vi "BT Rx Test Get Default Parameters.vi"(8 "error in (no error)":errorcluster, 11 "Rx Test in":refnum<class "niDTS BT Rx Test.lvclass">) -> (0 "error out":errorcluster, 2 "Parameters":T1={"Channel"=3, "Dut Tx Power"=0.0, "External Attenuation (dB)"=[0.0], "Data Rate"=enum."1", "Packet type"=enum."DH1", "Payload Data"=enum."PN9", "Carrier Mode"=enum."Burst", "Number of Packets"=1500, "Report Period (ms)"=1000.0, "BD ADDRESS"=0, "Dirty Tx"=FALSE, "Corrupt Alternate CRC"=FALSE, "Packet Header"={"LT Address"=0, "Flow"=0, "ARQN"=enum."NAK", "Sequence Bit"=0}, "Payload Header"={"LCh"=0, "HeaderFlowControlBit"=FALSE, "Length (-1 AutoSet Max)"=-1}, "Trigger"={"TriggerEdge"=enum."RISing", "TriggerSource"=enum."IMMediate", "TriggerDelay (sec)"=0.0, "TriggerTimeout (sec)"=0.0}} {"BD ADDRESS" max=16777215 format="%.0x"}, 3 "Rx Test out":refnum<class "niDTS BT Rx Test.lvclass">)   [LabVIEW 2015, in "niDTS BT.lvlib" / "niDTS BT Rx Test.lvclass"]
uses:
  niDTS BT Rx Test.lvclass
  Includes/niDTS BT Rx Test INC Parameters.ctl
  Includes/niDTS BT INC Packet Type.ctl
  Tx Test/Includes/niDTS BT Tx Test INC BD Payload Data.ctl
  Includes/niDTS BT Rx Test INC Carrier Mode.ctl
  Includes/niDTS BT Rx Test INC Packet Header.ctl
  Includes/niDTS BT Rx Test INC Payload Header.ctl
  Includes/niDTS BT DUT INC SG Trigger.ctl
  niDTS BT Rx Test.lvclass/niDTS BT Rx Test.ctl
  Includes/niDTS BT INC Standard.ctl
  niDTS BT.lvlib
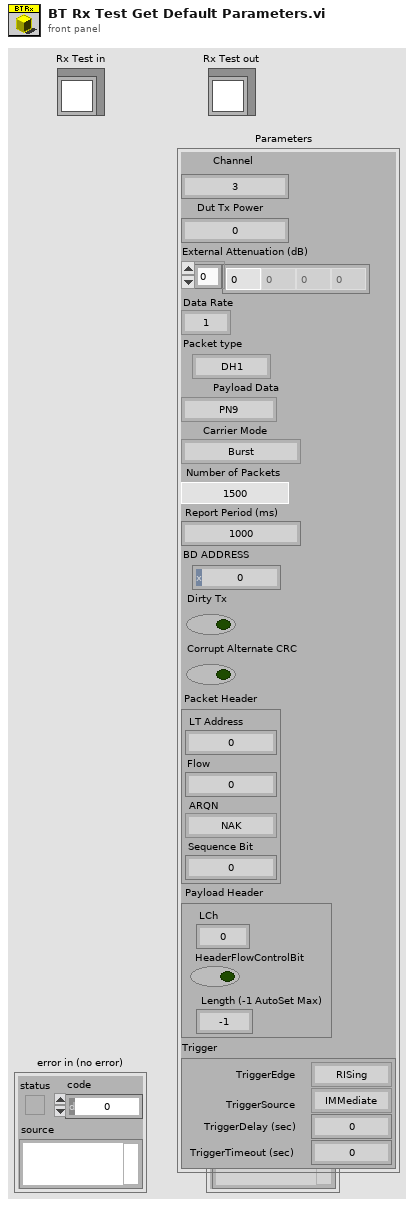
[diagram p1: front panel]
types:
  T1 = typedef "niDTS BT.lvlib/niDTS BT Rx Test INC Parameters.ctl" = cluster{"Channel":i32, "Dut Tx Power":dbl, "External Attenuation (dB)":dbl[], "Data Rate":enum16{"1", "2", "3"}, "Packet type":T2, "Payload Data":T3, "Carrier Mode":T4, "Number of Packets":i32, "Report Period (ms)":dbl, "BD ADDRESS":i64, "Dirty Tx":bool, "Corrupt Alternate CRC":bool, "Packet Header":T5, "Payload Header":T6, "Trigger":T7}
  T2 = typedef "niDTS BT.lvlib/niDTS BT INC Packet Type.ctl" = enum16{"NULL", "POLL", "FHS", "DM1", "DH1", "HV1", "HV2", "HV3", "EV3", "DV", "AUX1", "DM3", "DH3", "EV4", "EV5", "DM5", "DH5", "LE-TP"}
  T3 = typedef "niDTS BT.lvlib/niDTS BT Tx Test INC BD Payload Data.ctl" = enum16{"0", "1", "01", "00001111", "PN9", "AUTO"}
  T4 = typedef "niDTS BT.lvlib/niDTS BT Rx Test INC Carrier Mode.ctl" = enum16{"Burst", "Continuous"}
  T5 = typedef "niDTS BT.lvlib/niDTS BT Rx Test INC Packet Header.ctl" = cluster{"LT Address":i8, "Flow":i8, "ARQN":enum16{"NAK", "ACK"}, "Sequence Bit":i8}
  T6 = typedef "niDTS BT.lvlib/niDTS BT Rx Test INC Payload Header.ctl" = cluster{"LCh":i32, "HeaderFlowControlBit":bool, "Length (-1 AutoSet Max)":i32}
  T7 = typedef "niDTS BT.lvlib/niDTS BT DUT INC SG Trigger.ctl" = cluster{"TriggerEdge":enum16{"RISing", "FALLing"}, "TriggerSource":enum16{"IMMediate", "PFI 0", "PFI 1", "RTSI 0", "RTSI 1", "RTSI 2", "RTSI 3", "RTSI 4", "RTSI 5", "RTSI 6", "RTSI 7", "PXI STAR", "Software"}, "TriggerDelay (sec)":dbl, "TriggerTimeout (sec)":dbl}
  T8 = typedef "niDTS BT.lvlib/niDTS BT INC Standard.ctl" = enum16{"BDR", "EDR", "LE-TP"}
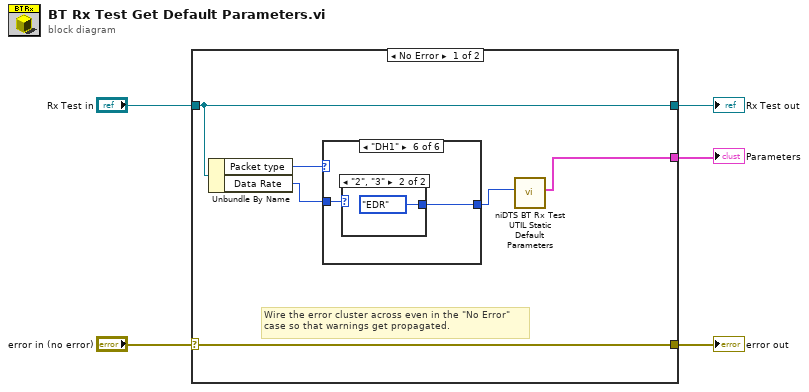
[diagram p0: block diagram]
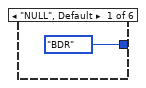
[diagram p2: hidden frame]
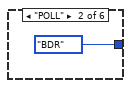
[diagram p3: hidden frame]
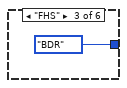
[diagram p4: hidden frame]
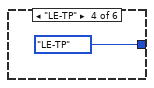
[diagram p5: hidden frame]
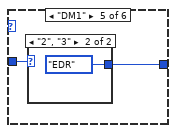
[diagram p6: hidden frame]
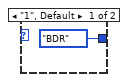
[diagram p7: hidden frame]
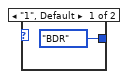
[diagram p8: hidden frame]
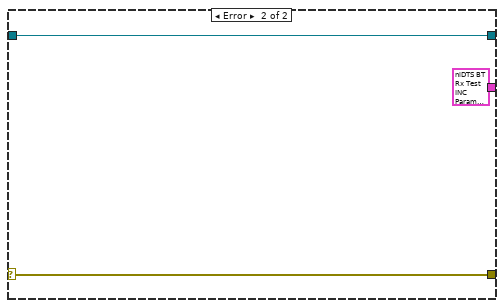
[diagram p9: hidden frame]
diagram:
  n1 = case shown="No Error" "error in (no error)" {
    selector: "error in (no error)" -> [w11 w26]
    tunnel: [w11 w26] -> w4
    tunnel: [w8 w25] -> w2
    tunnel: "Rx Test in" -> [w8 w25]
    tunnel: [w6 T1 {"Channel"=2, "Dut Tx Power"=7.0, "External Attenuation (dB)"=[0.0], "Data Rate"=enum."1", "Packet type"=enum."POLL", "Payload Data"=enum."00001111", "Carrier Mode"=enum."Continuous", "Number of Packets"=1500, "Report Period (ms)"=0.0, "BD ADDRESS"=12329017, "Dirty Tx"=FALSE, "Corrupt Alternate CRC"=FALSE, "Packet Header"={"LT Address"=0, "Flow"=0, "ARQN"=enum."NAK", "Sequence Bit"=0}, "Payload Header"={"LCh"=0, "HeaderFlowControlBit"=FALSE, "Length (-1 AutoSet Max)"=0}, "Trigger"={"TriggerEdge"=enum."RISing", "TriggerSource"=enum."IMMediate", "TriggerDelay (sec)"=0.0, "TriggerTimeout (sec)"=0.0}} ("Parameters")] -> w1
    frame No Error {
      # "Wire the error cluster across even in the \"No Error\"\ncase so that warnings get propagated."
      n2 = Unbundle By Name(w8) -> ("Packet type"=w10:T2, "Data Rate"=w9:enum16{"1", "2", "3"})
      n3 = case shown="\"DH1\"" w10 {
        tunnel: w9 -> [_ _ _ _ w17 w21]
        tunnel: [niDTS_BT_INC_Standard."BDR" ("BT Standard") niDTS_BT_INC_Standard."BDR" ("BT Standard") niDTS_BT_INC_Standard."BDR" ("BT Standard") niDTS_BT_INC_Standard."LE-TP" ("BT Standard") w16 w20] -> w7
        frame "NULL", Default {
        }
        frame "POLL" {
        }
        frame "FHS" {
        }
        frame "LE-TP" {
        }
        frame "DM1" {
          n4 = case shown="\"2\", \"3\"" w17 {
            tunnel: [niDTS_BT_INC_Standard."BDR" ("BT Standard") niDTS_BT_INC_Standard."EDR" ("BT Standard")] -> w16
            frame "1", Default {
            }
            frame "2", "3" {
            }
          }
        }
        frame "DH1" {
          n5 = case shown="\"2\", \"3\"" w21 {
            tunnel: [niDTS_BT_INC_Standard."BDR" ("BT Standard") niDTS_BT_INC_Standard."EDR" ("BT Standard")] -> w20
            frame "1", Default {
            }
            frame "2", "3" {
            }
          }
        }
      }
      n6 = call "niDTS BT Rx Test UTIL Static Default Parameters.vi"("BT Standard"=w7) -> ("Static Default Parameters"=w6:T1)  [unwired: 10 in]
    }
    frame Error {
    }
  }
  "error out" <- w4
  "Rx Test out" <- w2
  "Parameters" <- w1
